vi "Write vss_plays.vi"(8 "error in (no error)":errorcluster, 10 "vss_plays":T1, 11 "Playbook in":refnum<class "Playbook.lvclass">) -> (0 "error out":errorcluster, 3 "Playbook out":refnum<class "Playbook.lvclass">)   [LabVIEW 2023, in "Playbook.lvclass"]
uses:
  Playbook.lvclass
  PreparePenaltyAllyPlayVSS_class/PreparePenaltyAllyPlayVSS.lvclass
  HaltPlay_class/HaltPlay.lvclass
  DeadBallPlayVSS_class/DeadBallPlayVSS.lvclass
  NormalGamePlayVSS_class/NormalGamePlayVSS.lvclass
  BallChallengePlayVSS_class/BallChallengePlayVSS.lvclass
  PenaltyEnemyPlayVSS_class/PenaltyEnemyPlayVSS.lvclass
  TimeoutPlay_class/TimeoutPlay.lvclass
  KickPenaltyAllyPlayVSS_class/KickPenaltyAllyPlayVSS.lvclass
  PreparePenaltyEnemyPlayVSS_class/PreparePenaltyEnemyPlayVSS.lvclass
  PrepareKickoffAllyPlayVSS_class/PrepareKickoffAllyPlayVSS.lvclass
  PrepareKickoffEnemyPlayVSS_class/PrepareKickoffEnemyPlayVSS.lvclass
  PrepareGoalKickAllyPlayVSS_class/PrepareGoalKickAllyPlayVSS.lvclass
  PrepareGoalKickEnemyPlayVSS_class/PrepareGoalKickEnemyPlayVSS.lvclass
  PrepareFreeBallPlayVSS_class/PrepareFreeBallPlayVSS.lvclass
  FreeBallPlayVSS_class/FreeBallPlayVSS.lvclass
  GoalKickAllyPlayVSS_class/GoalKickAllyPlayVSS.lvclass
  GoalKickEnemyPlayVSS_class/GoalKickEnemyPlayVSS.lvclass
  KickoffAllyPlayVSS_class/KickoffAllyPlayVSS.lvclass
  KickoffEnemyPlayVSS_class/KickoffEnemyPlayVSS.lvclass
  StopPlayVSS_class/StopPlayVSS.lvclass
  Playbook.lvclass/Playbook.ctl
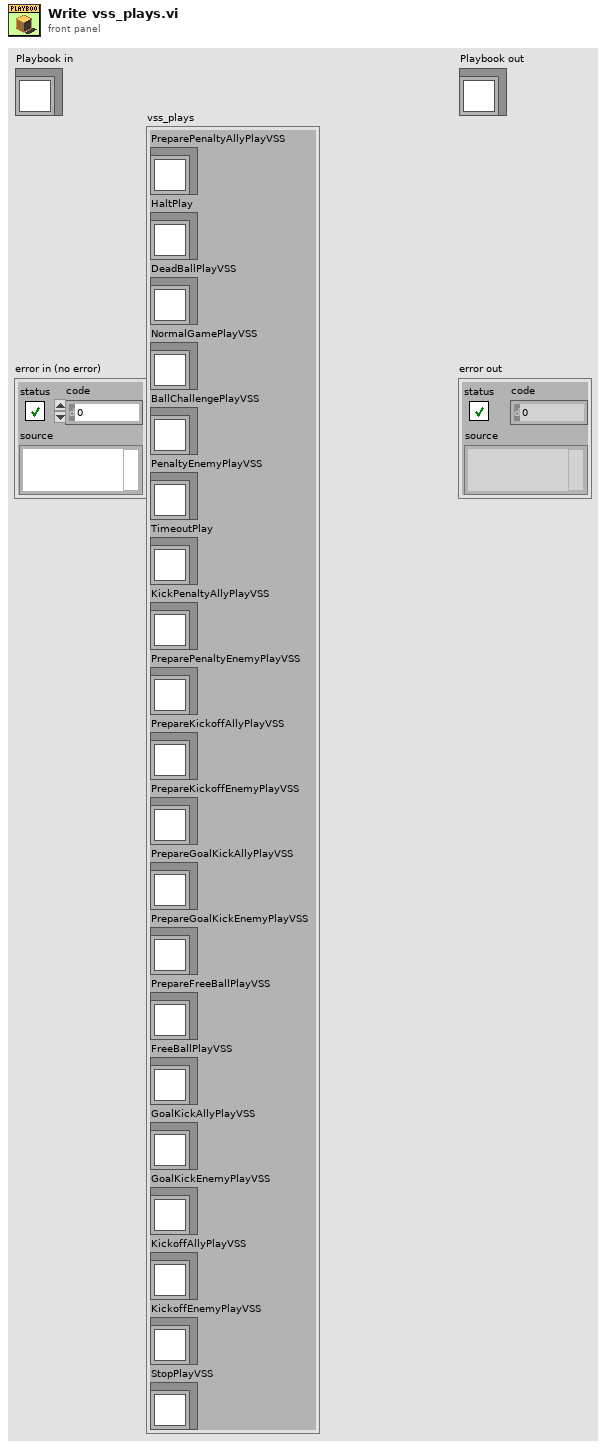
[diagram p1: front panel]
types:
  T1 = cluster{"PreparePenaltyAllyPlayVSS":refnum<class "PreparePenaltyAllyPlayVSS.lvclass">, "HaltPlay":refnum<class "HaltPlay.lvclass">, "DeadBallPlayVSS":refnum<class "DeadBallPlayVSS.lvclass">, "NormalGamePlayVSS":refnum<class "NormalGamePlayVSS.lvclass">, "BallChallengePlayVSS":refnum<class "BallChallengePlayVSS.lvclass">, "PenaltyEnemyPlayVSS":refnum<class "PenaltyEnemyPlayVSS.lvclass">, "TimeoutPlay":refnum<class "TimeoutPlay.lvclass">, "KickPenaltyAllyPlayVSS":refnum<class "KickPenaltyAllyPlayVSS.lvclass">, "PreparePenaltyEnemyPlayVSS":refnum<class "PreparePenaltyEnemyPlayVSS.lvclass">, "PrepareKickoffAllyPlayVSS":refnum<class "PrepareKickoffAllyPlayVSS.lvclass">, "PrepareKickoffEnemyPlayVSS":refnum<class "PrepareKickoffEnemyPlayVSS.lvclass">, "PrepareGoalKickAllyPlayVSS":refnum<class "PrepareGoalKickAllyPlayVSS.lvclass">, "PrepareGoalKickEnemyPlayVSS":refnum<class "PrepareGoalKickEnemyPlayVSS.lvclass">, "PrepareFreeBallPlayVSS":refnum<class "PrepareFreeBallPlayVSS.lvclass">, "FreeBallPlayVSS":refnum<class "FreeBallPlayVSS.lvclass">, "GoalKickAllyPlayVSS":refnum<class "GoalKickAllyPlayVSS.lvclass">, "GoalKickEnemyPlayVSS":refnum<class "GoalKickEnemyPlayVSS.lvclass">, "KickoffAllyPlayVSS":refnum<class "KickoffAllyPlayVSS.lvclass">, "KickoffEnemyPlayVSS":refnum<class "KickoffEnemyPlayVSS.lvclass">, "StopPlayVSS":refnum<class "StopPlayVSS.lvclass">}
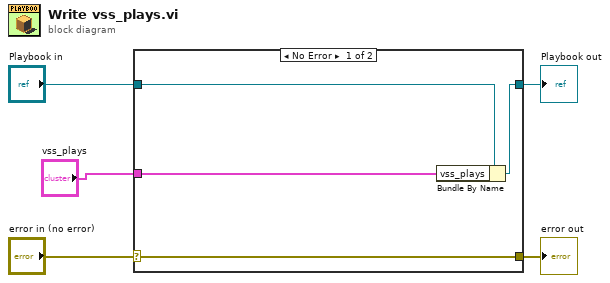
[diagram p0: block diagram]
diagram:
  n1 = case shown="No Error" "error in (no error)" {
    selector: "error in (no error)" -> [w9 w10]
    tunnel: [w9 w10] -> w4
    tunnel: [w7 w11] -> w2
    tunnel: "Playbook in" -> [w8 w11]
    tunnel: "vss_plays" -> [w6 _]
    frame No Error {
      n2 = Bundle By Name(cluster=w8, "vss_plays"=w6) -> (w7:refnum<class "Playbook.lvclass">)
    }
    frame Error {
    }
  }
  "error out" <- w4
  "Playbook out" <- w2
